vi "EstablishInheritence.vi"(8 "error in (no error)":errorcluster, 11 "ParseMermaid in":refnum<class "ParseMermaid.lvclass">) -> (0 "error out":errorcluster, 3 "ParseMermaid out":refnum<class "ParseMermaid.lvclass">)   [LabVIEW 2020, in "Mermaid.lvlib" / "ParseMermaid.lvclass"]
uses:
  ParseMermaid.lvclass
  ParseMermaid.lvclass/ParseMermaid.ctl
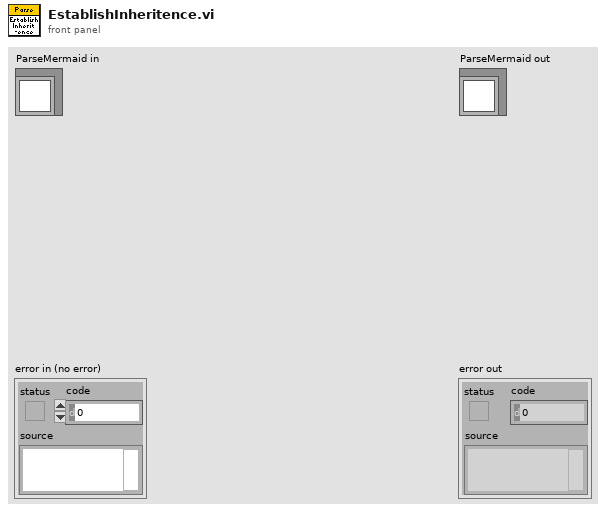
[diagram p1: front panel]
types:
  T1 = typedef "Mermaid.lvlib/ParseMermaid.lvclass/ClassData.ctl" = cluster{"Name":string, "ClassType":T2, "PublicMethods":string[], "PrivateMethods":string[], "FinalPublicAttributes":T3, "FinalPrivateAttributes":T3, "Parent":string}
  T2 = typedef "Mermaid.lvlib/ParseMermaid.lvclass/ClassType.ctl" = enum16{"Interface", "Class"}
  T3 = typedef "Mermaid.lvlib/ParseMermaid.lvclass/Attributes.ctl" = cluster{"Name":string, "Type":i32}[]
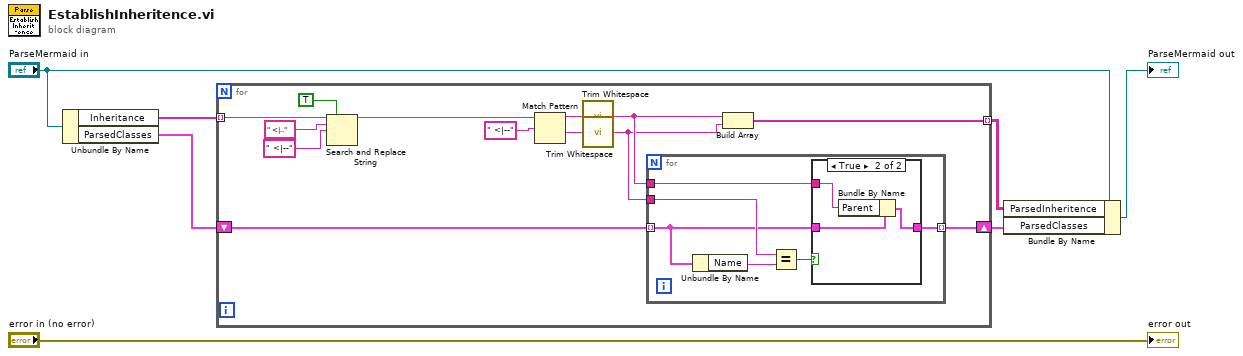
[diagram p0: block diagram]
diagram:
  n1 = Unbundle By Name("ParseMermaid in") -> ("Inheritance"=w5:string[], "ParsedClasses"=w6:T1[])
  n2 = for {
    tunnel: w5 -> [w12] mode=indexing
    shift-right: [w19] -> w4
    shift-left: w6 -> [w18]
    tunnel: [w13] -> w1 mode=indexing
    n3 = Search and Replace String(replace all?=TRUE ("replace all? (F)"), input string=w12, search string=" <|.." ("regular expression"), replace string=" <|--" ("regular expression")) -> (result string=w11:string)  [unwired: 4 in, 3 out]
    n4 = Match Pattern(string=w11, regular expression=" <|--") -> (before substring=w16:string, after substring=w17:string)  [unwired: 1 in, 2 out]
    n5 = call <vilib>:"Trim Whitespace.vi"("string"=w16) -> ("trimmed string"=w15:string)  [unwired: 1 in]
    n6 = call <vilib>:"Trim Whitespace.vi"("string"=w17) -> ("trimmed string"=w14:string)  [unwired: 1 in]
    n7 = for {
      tunnel: w18 -> [w24] mode=indexing
      tunnel: w14 -> [w25]
      tunnel: w15 -> [w23]
      tunnel: [w22] -> w19 mode=indexing
      n8 = Unbundle By Name(w24) -> ("Name"=w26:string)
      n9 = Equal?(x=w25, y=w26) -> (x = y?=w21:bool)
      n10 = case shown="True" w21 {
        tunnel: w24 -> [w27 w30]
        tunnel: w23 -> [_ w29]
        tunnel: [w27 w28] -> w22
        frame False {
        }
        frame True {
          n11 = Bundle By Name(cluster=w30, "Parent"=w29) -> (w28:T1)
        }
      }
    }
    n12 = Build Array(w15, w14) -> (w13:string[])
  }
  n13 = Bundle By Name(cluster="ParseMermaid in", "ParsedInheritence"=w1, "ParsedClasses"=w4) -> (→"ParseMermaid out":refnum<class "ParseMermaid.lvclass">)
  "error out" <- "error in (no error)"
